vi "HW_ni_DAQ.vi"(8 "error in":errorcluster caption="错误输入", 9 "daqModuPara[]":T2(array[cluster]), 10 "DeviceInfo":T3) -> (0 "error out":errorcluster caption="错误输出")   [LabVIEW 2016]
uses:
  Ctrls/Read and Write Ring.ctl
  <vilib>/DAQmx/create/channels.llb/DAQmx Create Channel (AI-Voltage-Basic).vi
  <vilib>/DAQmx/create/scale.llb/DAQmx Create Scale (Linear).vi
  <vilib>/DAQmx/read.llb/DAQmx Read (Analog 2D DBL NChan NSamp).vi
  <vilib>/DAQmx/configure/timing.llb/DAQmx Timing (Sample Clock).vi
  Ctrls/HardWare _ Data Queue Manage FGV Operation.ctl
  Ctrls/HardWare Basic Info _ Channel.ctl
  Ctrls/HardWare Basic Info _ Module.ctl
  Ctrls/HardWare Basic Info _ Chassis.ctl
  Ctrls/HardWare Basic Info _ Device.ctl
  Ctrls/HardWare _ Channel Parameters.ctl
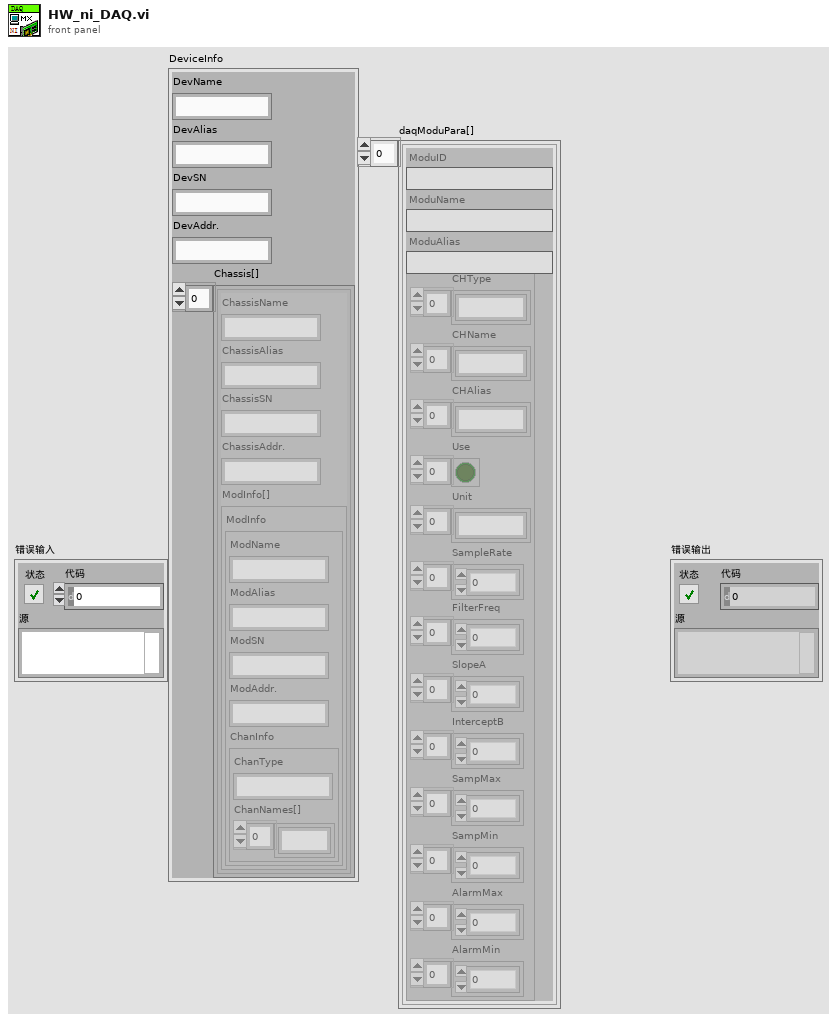
[diagram p1: front panel]
types:
  T1 = typedef "HardWare _ Channel Parameters.ctl" = cluster{"CHType":string[], "CHName":string[], "CHAlias":string[], "Use":bool[], "Unit":string[], "SampleRate":dbl[], "FilterFreq":dbl[], "SlopeA":dbl[], "InterceptB":dbl[], "SampMax":dbl[], "SampMin":dbl[], "AlarmMax":dbl[], "AlarmMin":dbl[]}
  T2 = cluster{"ModuID":string, "ModuName":string, "ModuAlias":string, "ChanPara":T1}[]
  T3 = typedef "HardWare Basic Info _ Device.ctl" = cluster{"DevName":string, "DevAlias":string, "DevSN":string, "DevAddr.":string, "Chassis[]":T4[]}
  T4 = typedef "HardWare Basic Info _ Chassis.ctl" = cluster{"ChassisName":string, "ChassisAlias":string, "ChassisSN":string, "ChassisAddr.":string, "ModInfo[]":T5[]}
  T5 = typedef "HardWare Basic Info _ Module.ctl" = cluster{"ModName":string, "ModAlias":string, "ModSN":string, "ModAddr.":string, "ChanInfo":T6}
  T6 = typedef "HardWare Basic Info _ Channel.ctl" = cluster{"ChanType":string, "ChanNames[]":string[]}
  T7 = typedef "HardWare _ Data Queue Manage FGV Operation.ctl" = enum16{"Initialize", "Add Chan", "Read Chan"}
  T8 = typedef "Read and Write Ring.ctl" = enum16{"Read", "Write"}
  T9 = typedef "HW_ni_Channel Configuration Structure.ctl" = cluster{"use":bool, "ChanName":string, "ChanAlias":string, "SampleRate":dbl, "SlopeA":dbl, "InterceptB":dbl, "Unit":string}
  T10 = cluster{i32, "data":dbl[][], dbl, "SampleRate":dbl}
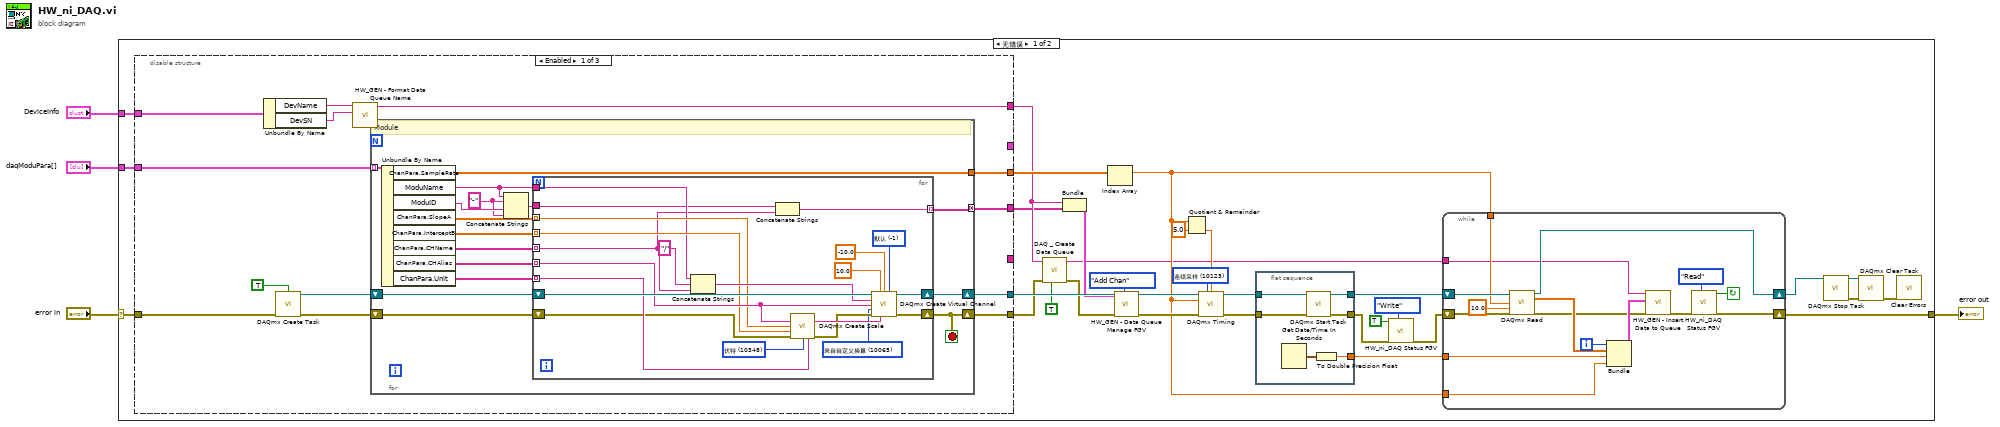
[diagram p0: block diagram]
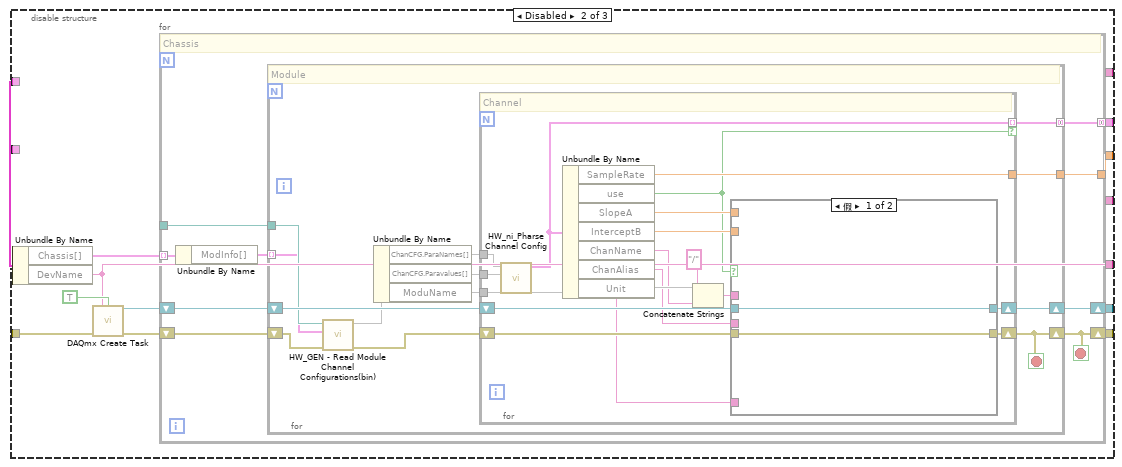
[diagram p2: hidden frame]
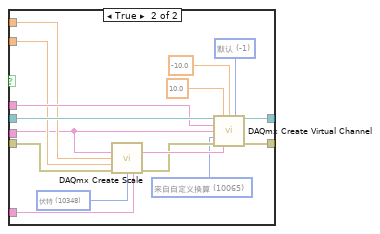
[diagram p3: hidden frame]
diagram:
  n1 = case shown="无错误" "error in" {
    selector: "error in" -> [w35 w177]
    tunnel: [w24 w177] -> w3
    tunnel: "DeviceInfo" -> [w34 _]
    tunnel: "daqModuPara[]" -> [w14 _]
    frame No Error {
      w33 = 10123 items=["有限采样"=10178, "连续采样"=10123, "硬件定时单点"=12522] ("sample mode")
      n2 = disable-structure shown="Disabled" {
        disable-tunnel: w35 -> [w48 w97 _]
        disable-tunnel: w34 -> [w46 w95 _]
        disable-tunnel: [w43 w90 _] -> w32
        disable-tunnel: [w42 w89 _] -> w27
        disable-tunnel: [_ w88 _] -> _
        disable-tunnel: [_ w87 _] -> _
        disable-tunnel: [w41 w86 _] -> w15
        disable-tunnel: w14 -> [w40 _ _]
        disable-tunnel: [w37 _ _] -> w12
        disable-tunnel: [w36 _ _] -> w11
        frame Enabled {
          n3 = Unbundle By Name(w46) -> ("DevName"=w39:string, "DevSN"=w38:string)
          n4 = call <vilib>:"DAQmx Create Task.vi"("auto cleanup"=TRUE, "error in"=w48) -> ("task out"=w45:refnum<k21>, "error out"=w44:errorcluster)  [unwired: 12 in]
          n5 = call "HW_GEN - Format Data Queue Name.vi"("DevSN"=w38, "DevName"=w39) -> ("Q Name"=w37:string)  [unwired: 9 in]
          n6 = for {
            shift-right: [w63] -> w43
            shift-left: w45 -> [w64]
            shift-right: [w62] -> w41
            shift-left: w44 -> [w60]
            tunnel: [w54] -> w42
            tunnel: w40 -> [w61] mode=indexing
            tunnel: [w49] -> w36 mode=concatenating
            stop <- w62 stop-if-true
            w51 = "-" ("string")
            # "Module"
            n7 = Unbundle By Name(w61) -> ("ChanPara.SampleRate"=w54:dbl[], "ModuName"=w53:string, "ModuID"=w52:string, "ChanPara.SlopeA"=w59:dbl[], "ChanPara.InterceptB"=w58:dbl[], "ChanPara.CHName"=w57:string[], "ChanPara.CHAlias"=w56:string[], "ChanPara.Unit"=w55:string[])
            n8 = Concatenate Strings(w53, w51, w52, w51) -> (w50:string)
            n9 = for {
              tunnel: w57 -> [w66] mode=indexing
              tunnel: w56 -> [w80] mode=indexing
              tunnel: w59 -> [w79] mode=indexing
              tunnel: w58 -> [w78] mode=indexing
              tunnel: w55 -> [w77] mode=indexing
              shift-right: [w84] -> w63
              shift-left: w64 -> [w85]
              shift-right: [w83] -> w62
              shift-left: w60 -> [w76]
              tunnel: w53 -> [w68]
              tunnel: w50 -> [w67]
              tunnel: [w65] -> w49 mode=indexing
              w69 = 10065 items=["伏特"=10348, "来自自定义换算"=10065] ("units")
              w72 = 10348 items=["伏特"=10348, "A"=10342, "Deg F"=10144, "Deg C"=10143, "Deg R"=10145, "开氏温标"=10325, "应变"=10299, "欧姆"=10384, "Hz"=10373, "秒"=10364, "米"=10219, "英寸"=10379, "度"=10146, "弧度"=10273, "时钟滴答"=10304, "g"=10186, "m/s^2"=12470, "m/s"=15959, "in/s"=15960, "帕"=10081, "Newtons"=15875, "Pounds"=15876, "kgf"=15877, "psi"=15879, "bar"=15880, "Nm"=15881, "oz-in"=15882, "lb-in"=15883, "lb-ft"=15884, "Volts/Volt"=15896, "mVolts/Volt"=15897, "来自TEDS"=12516] ("pre-scaled units")
              w73 = -1 items=["默认"=-1, "RSE"=10083, "NRSE"=10078, "差分"=10106, "伪差分"=12529] ("input terminal configuration")
              n10 = Concatenate Strings(w68, "/" ("字符串"), w66) -> (w82:string)
              n11 = Concatenate Strings(w67, w66) -> (w65:string)
              n12 = call-poly <vilib>:"DAQmx Create Scale.vi"("name"=w80, "slope"=w79, "y-intercept"=w78, "error in"=w76, "pre-scaled units"=w72, "scaled units"=w77) -> ("scale out"=w71:tag, "error out"=w70:errorcluster)  [unwired: 8 in]
              n13 = call-poly <vilib>:"DAQmx Create Virtual Channel.vi"("task in"=w85, "maximum value"=10.0, "minimum value"=-10.0, "input terminal configuration"=w73, "physical channels"=w82, "name to assign"=w80, "units"=w69, "error in"=w70, "custom scale name"=w71) -> ("task out"=w84:refnum<k21>, "error out"=w83:errorcluster)  [unwired: 5 in]
            }
          }
        }
        frame Disabled {
          n14 = Unbundle By Name(w95) -> ("Chassis[]"=w92:T4[], "DevName"=w87:string)
          n15 = call <vilib>:"DAQmx Create Task.vi"("new task name"=w87, "auto cleanup"=TRUE, "error in"=w97) -> ("task out"=w94:refnum<k21>, "error out"=w93:errorcluster)  [unwired: 11 in]
          n16 = for {
            shift-right: [w102] -> w90
            shift-left: w94 -> [w104]
            shift-right: [w101] -> w86
            shift-left: w93 -> [w103]
            tunnel: w92 -> [w106] mode=indexing
            tunnel: [w100] -> w91
            tunnel: [w99] -> w88 mode=concatenating
            tunnel: [w98] -> w89
            stop <- w101 stop-if-true
            # "Chassis"
            n17 = Unbundle By Name(w106) -> ("ModInfo[]"=w105:T5[])
            n18 = for {
              tunnel: w105 -> [w110] mode=indexing
              shift-right: [w118] -> w102
              shift-left: w104 -> [w119]
              shift-right: [w117] -> w101
              shift-left: w103 -> [w116]
              tunnel: w100 -> [w114]
              tunnel: [w109] -> w99 mode=concatenating
              tunnel: [w108] -> w98
              stop <- w117 stop-if-true
              # "Module"
              n19 = call "HW_GEN - Read Module Channel Configurations(bin).vi"("error in"=w116, 10:w110, "ModuCFG path"=w114) -> ("error out"=w115:errorcluster, 2:w113)  [unwired: 6 in, 1 out]
              n20 = Unbundle By Name(w113) -> ("ChanCFG.ParaNames[]"=w111, "ChanCFG.Paravalues[]"=w112, "ModuName"=w107)
              n21 = for {
                shift-right: [w135] -> w118
                shift-left: w119 -> [w136]
                shift-right: [w133] -> w117
                shift-left: w115 -> [w134]
                tunnel: w112 -> [w131]
                tunnel: w111 -> [w132]
                tunnel: [w130] -> w109 mode=indexing if=w120
                tunnel: [w129] -> w108
                tunnel: w107 -> [w128]
                # "Channel"
                n22 = call "HW_ni_Pharse Channel Config.vi"("Paravalues[]"=w131, "ParaNames[]"=w132) -> ("ChanCFG out"=w130:T9)  [unwired: 9 in]
                n23 = Unbundle By Name(w130) -> ("SampleRate"=w129:dbl, "use"=w120:bool, "SlopeA"=w123:dbl, "InterceptB"=w122:dbl, "ChanName"=w127:string, "ChanAlias"=w124:string, "Unit"=w121:string)
                n24 = Concatenate Strings(w128, "/" ("字符串"), w127) -> (w126:string)
                n25 = case shown="假" w120 {
                  tunnel: w136 -> [w137 w154]
                  tunnel: [w137 w153] -> w135
                  tunnel: w134 -> [w138 w147]
                  tunnel: [w138 w152] -> w133
                  tunnel: w126 -> [_ w148]
                  tunnel: w124 -> [_ w144]
                  tunnel: w123 -> [_ w146]
                  tunnel: w122 -> [_ w145]
                  tunnel: w121 -> [_ w142]
                  frame False {
                  }
                  frame True {
                    w139 = 10065 items=["伏特"=10348, "来自自定义换算"=10065] ("units")
                    w143 = 10348 items=["伏特"=10348, "A"=10342, "Deg F"=10144, "Deg C"=10143, "Deg R"=10145, "开氏温标"=10325, "应变"=10299, "欧姆"=10384, "Hz"=10373, "秒"=10364, "米"=10219, "英寸"=10379, "度"=10146, "弧度"=10273, "时钟滴答"=10304, "g"=10186, "m/s^2"=12470, "m/s"=15959, "in/s"=15960, "帕"=10081, "Newtons"=15875, "Pounds"=15876, "kgf"=15877, "psi"=15879, "bar"=15880, "Nm"=15881, "oz-in"=15882, "lb-in"=15883, "lb-ft"=15884, "Volts/Volt"=15896, "mVolts/Volt"=15897, "来自TEDS"=12516] ("pre-scaled units")
                    w149 = -1 items=["默认"=-1, "RSE"=10083, "NRSE"=10078, "差分"=10106, "伪差分"=12529] ("input terminal configuration")
                    n26 = call-poly <vilib>:"DAQmx Create Scale.vi"("name"=w144, "slope"=w146, "y-intercept"=w145, "error in"=w147, "pre-scaled units"=w143, "scaled units"=w142) -> ("scale out"=w141:tag, "error out"=w140:errorcluster)  [unwired: 8 in]
                    n27 = call-poly <vilib>:"DAQmx Create Virtual Channel.vi"("task in"=w154, "maximum value"=10.0, "minimum value"=-10.0, "input terminal configuration"=w149, "physical channels"=w148, "name to assign"=w144, "units"=w139, "error in"=w140, "custom scale name"=w141) -> ("task out"=w153:refnum<k21>, "error out"=w152:errorcluster)  [unwired: 5 in]
                  }
                }
              }
            }
          }
        }
        frame Disabled {
        }
      }
      n28 = call "DAQ _ Create Data Queue.vi"("如未找到则创建？(T)"=TRUE, "error in"=w15, "Q-name"=w12) -> ("error out"=w9:errorcluster, "queue name"=w5:string)  [unwired: 7 in]
      n29 = Bundle("Q Name"=w12, w11) -> (w10:cluster{"Q Name":string, string[]})  [unwired: 1 in]
      n30 = Index Array(array=w27) -> (element=w6:dbl)  [unwired: 1 in]
      n31 = call "HW_GEN - Data Queue Manage FGV.vi"("Oper."=HardWare___Data_Queue_Manage_FGV_Operation."Add Chan", "error in"=w9, "Add Chan"=w10) -> ("error out"=w8:errorcluster)  [unwired: 7 in, 1 out]
      n32 = Quotient & Remainder(x=w6, y=5.0) -> (floor(x/y)=w28:dbl)  [unwired: 1 out]
      n33 = call-poly <vilib>:"DAQmx Timing.vi"("task/channels in"=w32, "sample mode"=w33, "samples per channel"=w28, "rate"=w6, "error in"=w8) -> ("task out"=w31:refnum<k21>, "error out"=w29:errorcluster)  [unwired: 9 in]
      n34 = flat-sequence {
        tunnel: w31 -> [w160]
        tunnel: [w159] -> w30
        tunnel: w29 -> [w158]
        tunnel: [w157] -> w23
        tunnel: [w155] -> w25
        frame #0 {
          n35 = Get Date/Time In Seconds() -> (seconds since 1Jan1904=w156:timestamp)
          n36 = call <vilib>:"DAQmx Start Task.vi"("task/channels in"=w160, "error in"=w158) -> ("task out"=w159:refnum<k21>, "error out"=w157:errorcluster)  [unwired: 12 in]
          n37 = To Double Precision Float(number=w156) -> (double precision float=w155:dbl)
        }
      }
      n38 = call "HW_ni_DAQ Status FGV.vi"("Oper"=Read_and_Write_Ring."Write", "error in"=w23, "DAQ Status in"=TRUE) -> ("error out"=w22:errorcluster)  [unwired: 7 in, 1 out]
      n39 = while {
        shift-right: [w170] -> w19
        shift-left: w30 -> [w176]
        shift-right: [w167] -> w24
        shift-left: w22 -> [w175]
        tunnel: w6 -> [w174]
        tunnel: w25 -> [w171]
        tunnel: w6 -> [w165]
        tunnel: w5 -> [w163]
        i -> [w172]
        stop <- w168 continue-if-true
        n40 = call-poly <vilib>:"DAQmx Read.vi"("task/channels in"=w176, "number of samples per channel"=w174, "timeout"=10.0, "error in"=w175) -> ("task out"=w170:refnum<k21>, "data"=w166:dbl[][], "error out"=w162:errorcluster)  [unwired: 9 in]
        n41 = Bundle(w172, "data"=w166, w171, "SampleRate"=w165) -> (w164:T10)  [unwired: 1 in]
        n42 = call "HW_GEN - Insert Data to Queue.vi"("error in"=w162, "data"=w164, "Object Name"=w163) -> ("error out"=w161:errorcluster)  [unwired: 7 in, 1 out]
        n43 = call "HW_ni_DAQ Status FGV.vi"("Oper"=Read_and_Write_Ring."Read", "error in"=w161) -> ("error out"=w167:errorcluster, "DAQ Status out"=w168:bool)  [unwired: 8 in]
      }
      n44 = call <vilib>:"DAQmx Stop Task.vi"("task/channels in"=w19) -> ("task out"=w18:refnum<k21>, "error out"=w17:errorcluster)  [unwired: 13 in]
      n45 = call <vilib>:"DAQmx Clear Task.vi"("task in"=w18, "error in"=w17) -> ("error out"=w16:errorcluster)  [unwired: 13 in]
      n46 = call <vilib>:"Clear Errors.vi"("error in (no error)"=w16) -> ()  [unwired: 5 in, 2 out]
    }
    frame Error {
    }
  }
  "error out" <- w3
